vi "Response to Client.vi"(8 "error in (no error)":errorcluster, 9 "Context":variant, 10 "Message":variant, 11 "TCP Communications in":refnum<class "TCP Communications.lvclass">) -> (0 "error out":errorcluster, 1 "Context out":variant, 3 "TCP Communications out":refnum<class "TCP Communications.lvclass">)   [LabVIEW 2018, in "TCP Communications.lvclass"]
uses:
  TCP Communications.lvclass
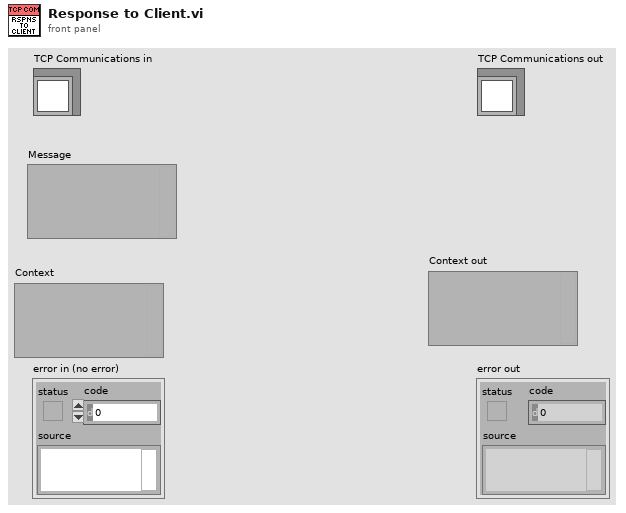
[diagram p1: front panel]
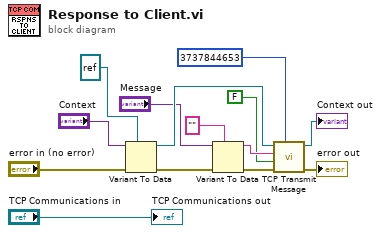
[diagram p0: block diagram]
diagram:
  n1 = Variant To Data(error in="error in (no error)", type=refnum<k5> refnum ("connection ID"), Variant="Context") -> (data=w12:refnum<k5>, error out=w11:errorcluster)
  n2 = Variant To Data(error in=w11, type="", Variant="Message") -> (data=w8:string, error out=w6:errorcluster)
  n3 = call "TCP Transmit Message.vi"("Magic"=u32 3737844653, "Error In"=w6, "Wait for response"=FALSE, "Message"=w8, "connection ID"=w12) -> ("Error Out"=→"error out":errorcluster, "connection ID out"=→"Context out":refnum<k5>)  [unwired: 3 in, 2 out]
  "TCP Communications out" <- "TCP Communications in"
